vi "oa_Check Averaging Parameters [OPS] (1 Channnel).vi"(6 "averaging parameters":T1={"averaging mode"=enum."No averaging", "weighting mode"=enum."Exponential", "number of averages"=10, "linear mode"=enum."One shot"} {"number of averages" min=1 step=1}, 8 "error in (no error)":errorcluster, 11 "resampled signal":cluster{"r0":dbl, "dr":dbl, "Y":dbl[]} {"r0" format="%.2p"; "dr" format="%.2p"; "Y" format="%.2f"}) -> (0 "error out":errorcluster, 2 "parameter changed":bool, 3 "resampled signal dup":cluster{"r0":dbl, "dr":dbl, "Y":dbl[]} {"r0" format="%.2p"; "dr" format="%.2p"; "Y" format="%.2f"})   [LabVIEW 2017, in "SoundVib_Resampling.lvlib"]
uses:
  <vilib>/addons/Sound and Vibration/Order Analysis/Resample Order Tracking/SoundVib_Resampling.lvlib
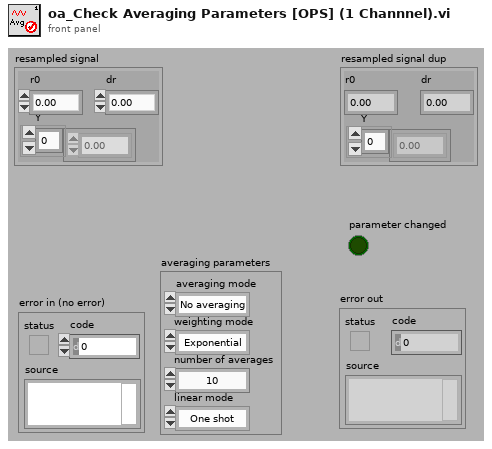
[diagram p1: front panel]
types:
  T1 = cluster{"averaging mode":enum16{"No averaging", "Vector averaging", "RMS averaging", "Peak hold"}, "weighting mode":enum16{"Linear", "Exponential"}, "number of averages":u32, "linear mode":enum16{"One shot", "Auto restart"}}
  T2 = enum16{"No averaging", "Vector averaging", "RMS averaging", "Peak hold"}
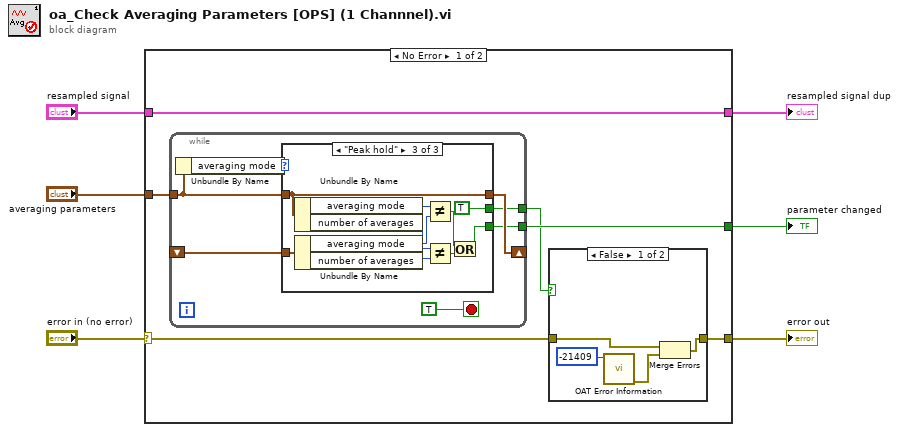
[diagram p0: block diagram]
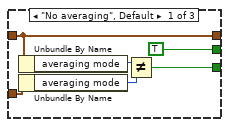
[diagram p3: hidden frame]
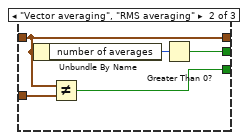
[diagram p4: hidden frame]
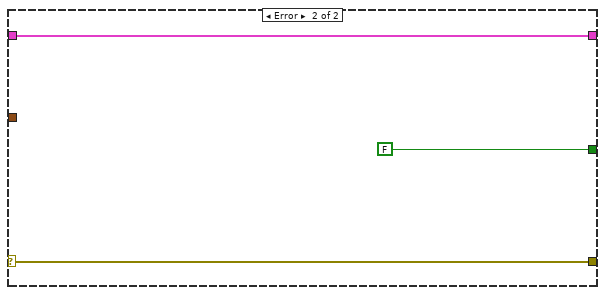
[diagram p5: hidden frame]
diagram:
  n1 = case shown="No Error" "error in (no error)" {
    selector: "error in (no error)" -> [w8 w48]
    tunnel: [w7 w48] -> w5
    tunnel: "resampled signal" -> [w12 w47]
    tunnel: [w12 w47] -> w3
    tunnel: "averaging parameters" -> [w11 _]
    tunnel: [w10 FALSE] -> w1
    frame No Error {
      n2 = while {
        tunnel: w11 -> [w22]
        shift-right: [w21] -> _
        shift-left: _ -> [w20]
        tunnel: [w19] -> w10
        tunnel: [w18] -> w9
        stop <- TRUE stop-if-true
        n3 = Unbundle By Name(w22) -> ("averaging mode"=w23:T2)
        n4 = case shown="\"Peak hold\"" w23 {
          tunnel: w22 -> [w30 w33 w45]
          tunnel: [w30 w33 w45] -> w21
          tunnel: w20 -> [w29 w34 w44]
          tunnel: [w26 w32 w37] -> w19
          tunnel: [TRUE w31 TRUE] -> w18
          frame "No averaging", Default {
            n5 = Unbundle By Name(w30) -> ("averaging mode"=w28:T2)
            n6 = Unbundle By Name(w29) -> ("averaging mode"=w27:T2)
            n7 = Not Equal?(x=w28, y=w27) -> (x != y?=w26:bool)
          }
          frame "Vector averaging", "RMS averaging" {
            n8 = Unbundle By Name(w33) -> ("number of averages"=w35:u32)
            n9 = Not Equal?(x=w33, y=w34) -> (x != y?=w32:bool)
            n10 = Greater Than 0?(x=w35) -> (x > 0?=w31:bool)
          }
          frame "Peak hold" {
            n11 = Unbundle By Name(w45) -> ("averaging mode"=w43:T2, "number of averages"=w40:u32)
            n12 = Unbundle By Name(w44) -> ("averaging mode"=w42:T2, "number of averages"=w41:u32)
            n13 = Not Equal?(x=w43, y=w42) -> (x != y?=w38:bool)
            n14 = Not Equal?(x=w40, y=w41) -> (x != y?=w39:bool)
            n15 = Or(x=w38, y=w39) -> (x .or. y?=w37:bool)
          }
        }
      }
      n16 = case shown="False" w9 {
        tunnel: w8 -> [w15 w17]
        tunnel: [w13 w17] -> w7
        frame False {
          n17 = call <vilib>:"OAT Error Information.vi"("error code"=-21409) -> ("error out"=w14:errorcluster)  [unwired: 6 in]
          n18 = Merge Errors(w15, w14) -> (w13:errorcluster)
        }
        frame True {
        }
      }
    }
    frame Error {
    }
  }
  "resampled signal dup" <- w3
  "error out" <- w5
  "parameter changed" <- w1
